vi "Read DMM Setting.vi"(8 "error in (no error)":errorcluster, 11 "DMM configuration in":refnum<class "DMM configuration.lvclass">) -> (0 "error out":errorcluster, 2 "DMM Setting":T1={"Function"="DC Volts", "CurrentSource"="1mA", "Resolution"="5 1/2", "Range"=0.5} {"Range" format="%#_f"}, 3 "DMM configuration out":refnum<class "DMM configuration.lvclass">)   [LabVIEW 2025, in "DMM.lvlib" / "DMM configuration.lvclass"]
uses:
  DMM configuration.lvclass
  DMM Setting.ctl
  DMM configuration.lvclass/DMM configuration.ctl
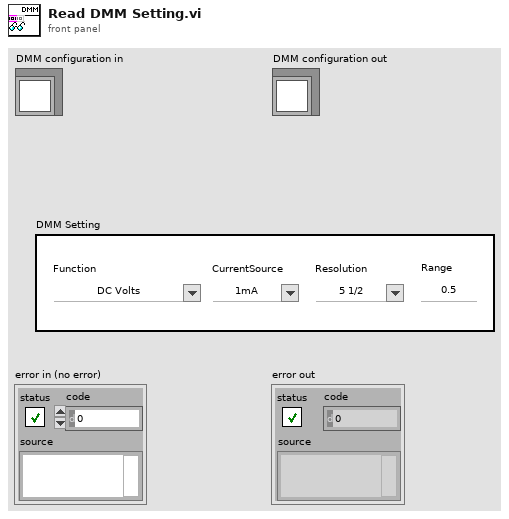
[diagram p1: front panel]
types:
  T1 = typedef "DMM.lvlib/DMM configuration.lvclass/DMM Setting.ctl" = cluster{"Function":string, "CurrentSource":string, "Resolution":string, "Range":dbl}
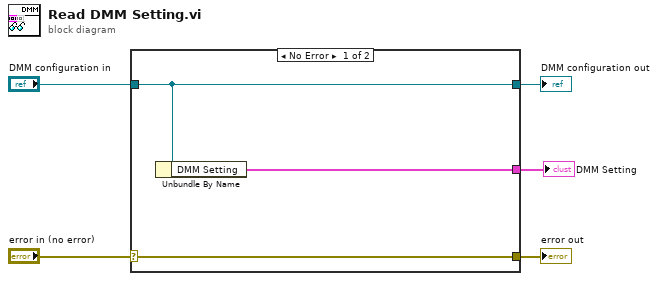
[diagram p0: block diagram]
diagram:
  n1 = case shown="No Error" "error in (no error)" {
    selector: "error in (no error)" -> [w8 w9]
    tunnel: [w8 w9] -> w4
    tunnel: [w7 w10] -> w2
    tunnel: "DMM configuration in" -> [w7 w10]
    tunnel: [w6 _] -> w1
    frame No Error {
      n2 = Unbundle By Name(w7) -> ("DMM Setting"=w6:T1)
    }
    frame Error {
    }
  }
  "error out" <- w4
  "DMM configuration out" <- w2
  "DMM Setting" <- w1
